vi "PR_check_barcode.vi"(7 "Boolean":bool, 8 "error in (no error)":errorcluster, 9 "Barcode_B":string, 10 "Barcode_A":string, 11 "DBlink":string="Driver={ODBC Driver 17 for SQL Server};Server=localhost\\SQLEXPRESS;Database=ZDX201;UID=labview;PWD=Dsa@54137926") -> (0 "error out":errorcluster, 1 "data":cluster{string}[](array[cluster]), 2 "是否為新資料":bool)   [LabVIEW 2019]
uses:
  <vilib>/addons/database/Connection.llb/DB Tools Open Connec (String).vi
  <vilib>/addons/database/Connection.llb/Conn Execute.vi
  <vilib>/addons/database/Recordset.llb/Rec Fetch Recordset Data (R).vi
  <vilib>/addons/database/Recordset.llb/Rec Destroy - Connection.vi
  <vilib>/addons/database/_DB Variant To Data/Database Variant To Data.xnode
  <vilib>/addons/database/NI_Database_API.lvlib
panel:
  out "Command 1":string="SELECT TOP (1) [id]      \n FROM [ZDX201].[dbo].[glue_data]\n where glue_workspace_id=4\nand evaluation_1 is null\norder by id desc "
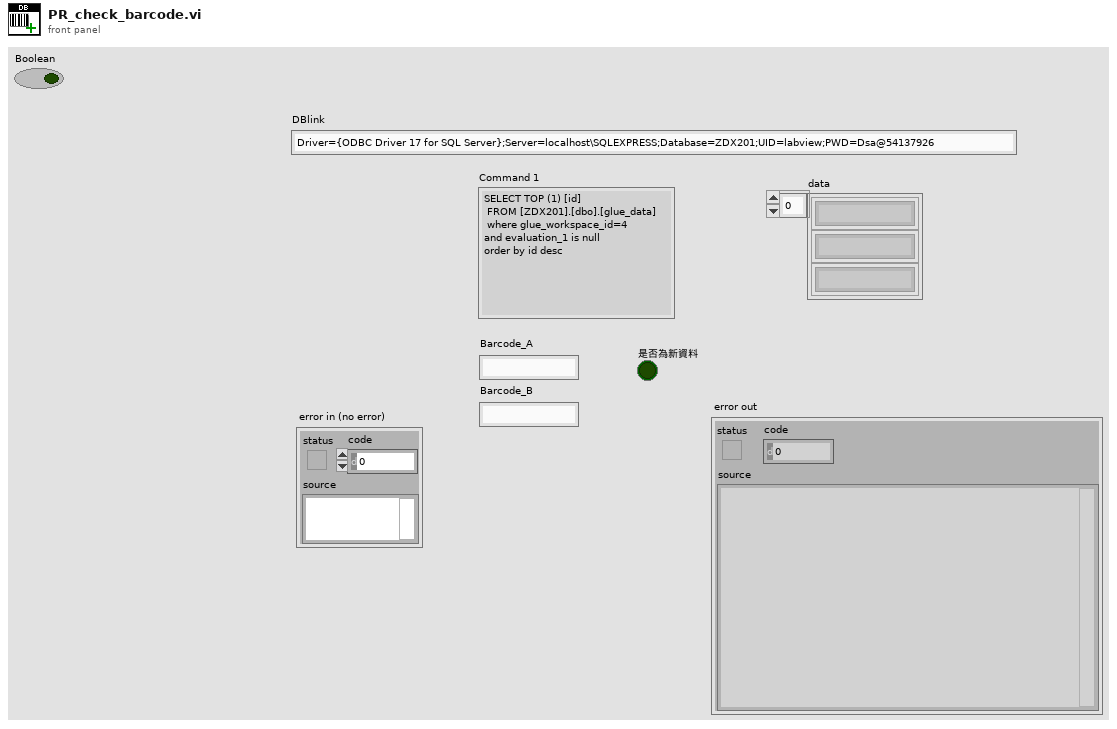
[diagram p1: front panel]
types:
  T1 = typedef "NI_Database_API.lvlib/Conn ObjectReference.ctl" = refnum<k1>
  T2 = typedef "NI_Database_API.lvlib/Rec ObjectReference.ctl" = refnum<k1>
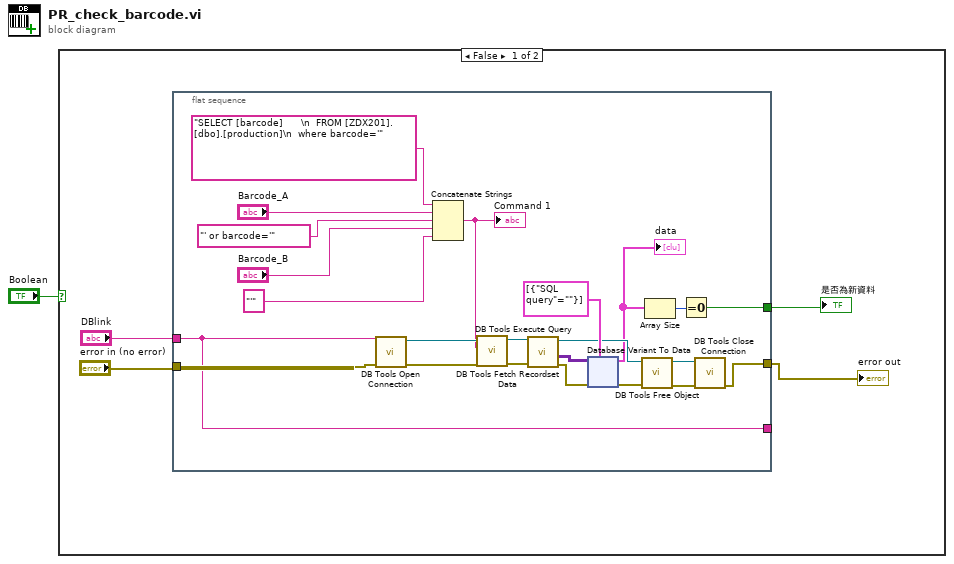
[diagram p0: block diagram]
diagram:
  n1 = case shown="False" "Boolean" {
    frame False {
      n2 = flat-sequence {
        tunnel: "DBlink" -> [w16]
        tunnel: "error in (no error)" -> [w28]
        tunnel: [w17] -> w3
        tunnel: [w16] -> _
        tunnel: [w6] -> w2
        frame #0 {
          n3 = call-poly <vilib>:"DB Tools Open Connection.vi"("error in (no error)"=w28, "connection information"=w16) -> ("error out"=w27:errorcluster, "connection reference"=w26:T1)  [unwired: 6 in]
          n4 = Concatenate Strings("SELECT [barcode]      \n  FROM [ZDX201].[dbo].[production]\n  where barcode='" ("SQL query"), "Barcode_A", "' or barcode='" ("SQL query"), "Barcode_B", "'" ("SQL query")) -> (w9:string)
          "Command 1" <- w9
          n5 = call-poly <vilib>:"DB Tools Execute Query.vi"("error in (no error)"=w27, "SQL query"=w9, "connection reference"=w26) -> ("error out"=w25:errorcluster, "recordset reference"=w24:T2)  [unwired: 5 in]
          n6 = call-poly <vilib>:"DB Tools Fetch Recordset Data.vi"("error in (no error)"=w25, "recordset reference"=w24) -> ("error out"=w23:errorcluster, "recordset data"=w15:variant[][], "recordset reference out"=w18:T2)  [unwired: 3 in]
          n7 = xnode "Database Variant To Data"("database variant"=w15, "error in (no error)"=w23, "type"=cluster{"SQL query":string}[] [{"SQL query"=""}] ("initialized array")) -> ("data"=w8:cluster{"SQL query":string}[], "error out"=w19:errorcluster)
          "data" <- w8
          n8 = call-poly <vilib>:"DB Tools Free Object.vi"("error in (no error)"=w19, "recordset reference"=w18) -> ("error out"=w20:errorcluster, "connection reference"=w21:T1)  [unwired: 8 in]
          n9 = Array Size(array=w8) -> (size(s)=w7:i32)
          n10 = Equal To 0?(x=w7) -> (x = 0?=w6:bool)
          n11 = call <vilib>:"DB Tools Close Connection.vi"("error in (no error)"=w20, "connection reference"=w21) -> ("error out"=w17:errorcluster)  [unwired: 5 in]
        }
      }
      "error out" <- w3
      "是否為新資料" <- w2
    }
    frame True {
    }
  }
